vi "Parse File Info Row.vi"(11 "File Info":T1) -> (3 "Column Fields":string[](array[string]))   [LabVIEW 2020, in "Peer Review.lvclass"]
uses:
  Peer Review.lvclass
  TypeDefs/File Info.ctl
  TypeDefs/File State.ctl
  TypeDefs/VI Type.ctl
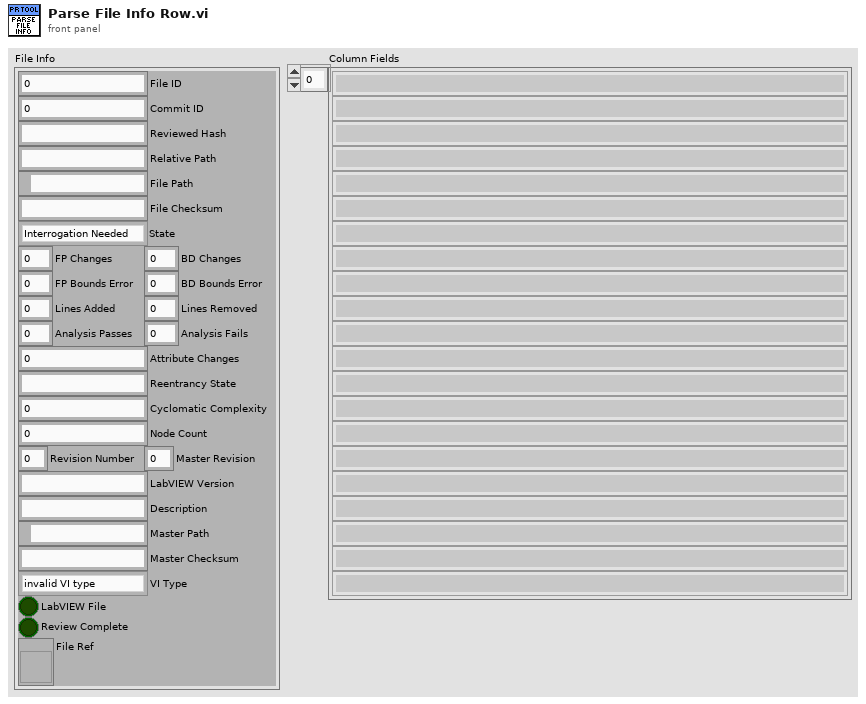
[diagram p1: front panel]
types:
  T1 = typedef "Peer Review.lvclass/File Info.ctl" = cluster{"File ID":i32, "Commit ID":i32, "Reviewed Hash":string, "Relative Path":string, "File Path":path, "File Checksum":string, "State":T2, "FP Changes":i32, "BD Changes":i32, "FP Bounds Error":dbl, "BD Bounds Error":dbl, "Lines Added":i32, "Lines Removed":i32, "Analysis Passes":i32, "Analysis Fails":i32, "Attribute Changes":i32, "Reentrancy State":string, "Cyclomatic Complexity":i32, "Node Count":i32, "Revision Number":u32, "LabVIEW Version":string, "Description":string, "Master Path":path, "Master Checksum":string, "VI Type":T3, "LabVIEW File":bool, "Review Complete":bool, "File Ref":refnum<vi>, "Master Revision":u32}
  T2 = typedef "Peer Review.lvclass/File State.ctl" = enum16{"Interrogation Needed", "Modified", "Deleted", "Added", "Matches Previous", "No Changes", "Moved", "Empty File"}
  T3 = typedef "Peer Review.lvclass/VI Type.ctl" = enum32{"invalid VI type", "Standard VI", "Control VI", "Global VI", "Polymorphic VI", "Configuration VI", "SubSystem", "Facade VI", "Method VI", "Statechart Diagram VI"}
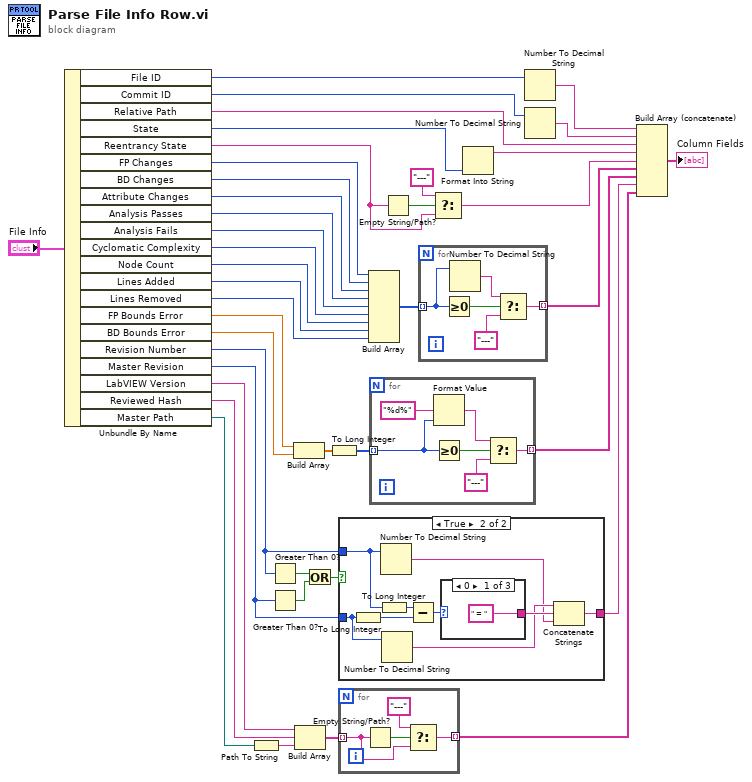
[diagram p0: block diagram]
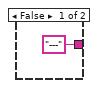
[diagram p2: hidden frame]
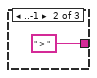
[diagram p3: hidden frame]
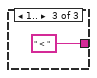
[diagram p4: hidden frame]
diagram:
  n1 = Unbundle By Name("File Info") -> ("File ID"=w39:i32, "Commit ID"=w37:i32, "Relative Path"=w40:string, "State"=w34:T2, "Reentrancy State"=w23:string, "FP Changes"=w29:i32, "BD Changes"=w31:i32, "Attribute Changes"=w30:i32, "Analysis Passes"=w27:i32, "Analysis Fails"=w26:i32, "Cyclomatic Complexity"=w20:i32, "Node Count"=w19:i32, "Lines Added"=w18:i32, "Lines Removed"=w17:i32, "FP Bounds Error"=w11:dbl, "BD Bounds Error"=w10:dbl, "Revision Number"=w6:u32, "Master Revision"=w4:u32, "LabVIEW Version"=w12:string, "Reviewed Hash"=w14:string, "Master Path"=w33:path)
  n2 = Path To String(path=w33) -> (string=w16:string)
  n3 = Greater Than 0?(x=w6) -> (x > 0?=w3:bool)
  n4 = Greater Than 0?(x=w4) -> (x > 0?=w2:bool)
  n5 = Build Array(w11, w10) -> (w9:dbl[])
  n6 = Build Array(w12, w14, w16) -> (w15:string[])
  n7 = Or(x=w3, y=w2) -> (x .or. y?=w1:bool)
  n8 = To Long Integer(number=w9) -> (32bit integer=w7:i32[])
  n9 = case shown="True" w1 {
    tunnel: w6 -> [_ w46]
    tunnel: ["---" w47] -> w5
    tunnel: w4 -> [_ w45]
    frame False {
    }
    frame True {
      n10 = To Long Integer(number=w45) -> (32bit integer=w50:i32)
      n11 = To Long Integer(number=w46) -> (32bit integer=w51:i32)
      n12 = Number To Decimal String(number=w46) -> (decimal integer string=w43:string)  [unwired: 1 in]
      n13 = Number To Decimal String(number=w45) -> (decimal integer string=w44:string)  [unwired: 1 in]
      n14 = Subtract(x=w51, y=w50) -> (x-y=w49:i32)
      n15 = case shown="0" w49 {
        tunnel: [" = " " > " " < "] -> w48
        frame 0 {
        }
        frame ..-1 {
        }
        frame 1.. {
        }
      }
      n16 = Concatenate Strings(w44, w48, w43) -> (w47:string)
    }
  }
  n17 = for {
    tunnel: [w58] -> w13 mode=indexing
    tunnel: w15 -> [w56] mode=indexing
    n18 = Empty String/Path?(string/path=w56) -> (empty?=w57:bool)
    n19 = Select(t="---" ("element"), s=w57, f=w56) -> (s? t:f=w58:string)
  }
  n20 = Build Array(w29, w31, w30, w27, w26, w20, w19, w18, w17) -> (w28:i32[])
  n21 = for {
    tunnel: w7 -> [w60] mode=indexing
    tunnel: [w62] -> w8 mode=indexing
    n22 = Format Value(format string="%d%", value (0)=w60) -> (output string=w59:string)  [unwired: 1 in]
    n23 = Greater Or Equal To 0?(x=w60) -> (x >= 0?=w63:bool)
    n24 = Select(t=w59, s=w63, f="---" ("element")) -> (s? t:f=w62:string)
  }
  n25 = Empty String/Path?(string/path=w23) -> (empty?=w25:bool)
  n26 = for {
    tunnel: [w67] -> w32 mode=indexing
    tunnel: w28 -> [w65] mode=indexing
    n27 = Greater Or Equal To 0?(x=w65) -> (x >= 0?=w69:bool)
    n28 = Number To Decimal String(number=w65) -> (decimal integer string=w68:string)  [unwired: 1 in]
    n29 = Select(t=w68, s=w69, f="---" ("element")) -> (s? t:f=w67:string)
  }
  n30 = Select(t="---", s=w25, f=w23) -> (s? t:f=w22:string)
  n31 = Format Into String(w34) -> (resulting string=w35:string)  [unwired: 3 in, 1 out]
  n32 = Number To Decimal String(number=w39) -> (decimal integer string=w38:string)  [unwired: 1 in]
  n33 = Number To Decimal String(number=w37) -> (decimal integer string=w36:string)  [unwired: 1 in]
  n34 = Build Array (concatenate)(w38, w36, w40, w35, w22, w32, w8, w5, w13) -> (→"Column Fields":string[])
